vi "Write Blink.vi"(8 "error in (no error)":errorcluster, 9 "Blink On":bool, 10 "Session In":refnum<class "Session.lvclass">, 11 "Grove I2C LCD I in":refnum<class "Grove I2C LCD.lvclass">) -> (0 "error out":errorcluster, 2 "Session Out":refnum<class "Session.lvclass">, 3 "Grove I2C LCD I out":refnum<class "Grove I2C LCD.lvclass">)   [LabVIEW 2020, in "CTI-Peripheral.lvlib" / "Grove I2C LCD.lvclass"]
uses:
  Grove I2C LCD.lvclass
  CTI/Session/Session.lvclass
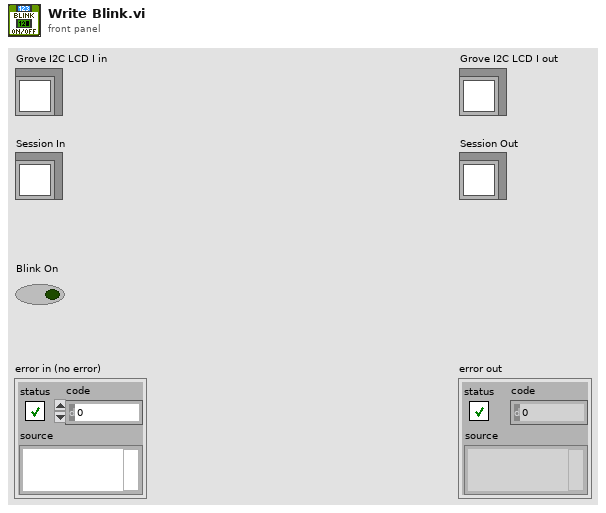
[diagram p1: front panel]
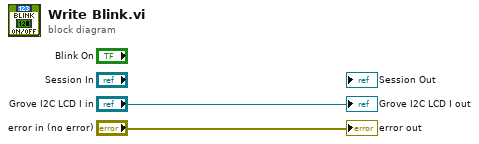
[diagram p0: block diagram]
diagram:
  "error out" <- "error in (no error)"
  "Grove I2C LCD I out" <- "Grove I2C LCD I in"
